vi "Selected Item Callback.vi"(4 "Net Event Data":T1, 5 "Event Data":cluster{"selectedItem":T2}, 6 "Control Ref":T3, 7 "Event Common Data":T4) -> ()   [LabVIEW 2020, in "NI_VS UI Single Node Browser.lvlib"]
uses:
  <vilib>/NI VeriStand/UI Controls/Single Node Browser/NI_VS UI Single Node Browser.lvlib
  <vilib>/NI VeriStand/UI Controls/Single Node Browser/Single Node Browser Ref.ctl
  NationalInstruments.VeriStand.SystemStorageUI
  <vilib>/NI VeriStand/UI Controls/Single Node Browser/Node Ref.ctl
  NationalInstruments.VeriStand.SystemStorage
  <vilib>/NI VeriStand/UI Controls/Single Node Browser/Net Event Data Ref.ctl
  <vilib>/NI VeriStand/UI Controls/Single Node Browser/Net Event Data.ctl
  <vilib>/NI VeriStand/UI Controls/Single Node Browser/Net Event.ctl
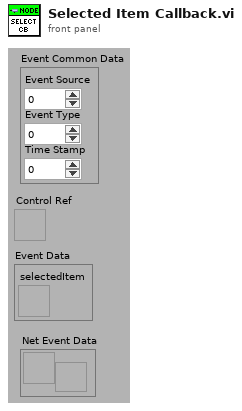
[diagram p1: front panel]
types:
  T1 = typedef "NI_VS UI Single Node Browser.lvlib/Net Event Data Ref.ctl" = refnum<user-event>
  T2 = typedef "NI_VS UI Single Node Browser.lvlib/Node Ref.ctl" = refnum<k24>
  T3 = typedef "NI_VS UI Single Node Browser.lvlib/Single Node Browser Ref.ctl" = refnum<k24>
  T4 = cluster{"Event Source":i32, "Event Type":u32, "Time Stamp":u32}
  T5 = typedef "NI_VS UI Single Node Browser.lvlib/Net Event Data.ctl" = cluster{"Event":T6, "Data":variant}
  T6 = typedef "NI_VS UI Single Node Browser.lvlib/Net Event.ctl" = enum16{"SelectedItem"}
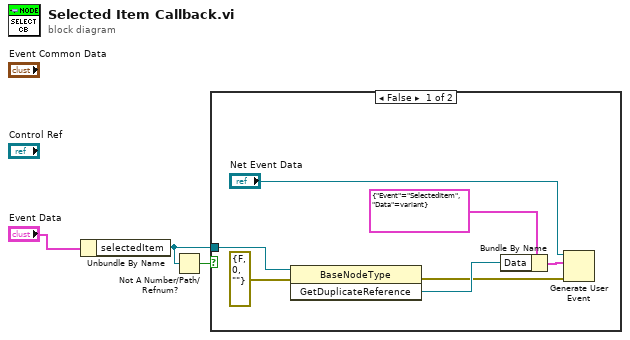
[diagram p0: block diagram]
diagram:
  n1 = Unbundle By Name("Event Data") -> ("selectedItem"=w3:T2)
  n2 = Not A Number/Path/Refnum?(number/path/refnum=w3) -> (NaN/Path/Refnum?=w2:bool)
  n3 = case shown="False" w2 {
    tunnel: w3 -> [w7 _]
    frame False {
      n4 = invoke class="BaseNodeType" method="GetDuplicateReference"(reference=w7, error in=errorcluster {"status"=FALSE, "code"=0, "source"=""} ("error out")) -> (error out=w4:errorcluster, "GetDuplicateReference"=w5:refnum<k24>)  [unwired: 1 in, 1 out]
      n5 = Bundle By Name(cluster=T5 {"Event"=enum."SelectedItem", "Data"=variant} ("event data"), "Data"=w5) -> (w9:T5)
      n6 = Generate User Event(user event="Net Event Data", event data cluster=w9, error in=w4) -> ()  [unwired: 1 in, 2 out]
    }
    frame True {
    }
  }
